vi "GetLevelButtons.vi"(10 "Control Box":bool[](array[boolean])) -> (2 "Level Buttons":bool[](array[boolean]))   [LabVIEW 2014]
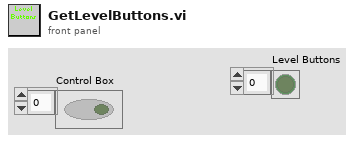
[diagram p1: front panel]
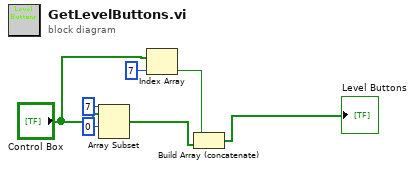
[diagram p0: block diagram]
diagram:
  n1 = Array Subset(array="Control Box", index=0, length=7) -> (w5:bool[])
  n2 = Index Array(array="Control Box", index=7) -> (element=w2:bool)
  n3 = Build Array (concatenate)(w2, w5) -> (→"Level Buttons":bool[])
